vi "GlobalIODataSize7.vi"() -> ()   [LabVIEW 2013]
panel:
  in  "IODataSize":i32=2048
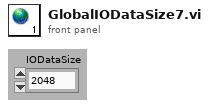
[diagram p1: front panel]
diagram:
